vi "WPI_Power Get 3Volt Rail Voltage and Current.vi"(11 "error in":errorcluster) -> (6 "3.3 volt rail voltage (V)":dbl, 8 "3.3 volt rail current (A)":dbl, 15 "error out":errorcluster)   [LabVIEW 2017]
doc: "Returns the voltage and current of the 3.3 volt user rail on the roboRIO in the robot program. On the roboRIO the 3.3 volt rail is connected to:\npin V of DIO channels (internal jumper set to 3.3V)\npin 3.3V of SPI\npin 3.3V of I2C\npin 33 of MXP"
uses:
  <vilib>/Utility/error.llb/Error Cluster From Error Code.vi
  <vilib>/rvi/errors/niLvFpgaAdjustHostInterfaceError.vi
  <vilib>/rvi/interface/nirviReadWriteControl/nirviReadWriteControl.xnode
  <vilib>/Rock Robotics/SystemInterfaces/System/FPGA_SystemFRC FPGA Ref.ctl
  NiFpgaLv.dll
  <vilib>/rvi/interface/Simulation/niFpgaSimulationCallBeginRW.vi
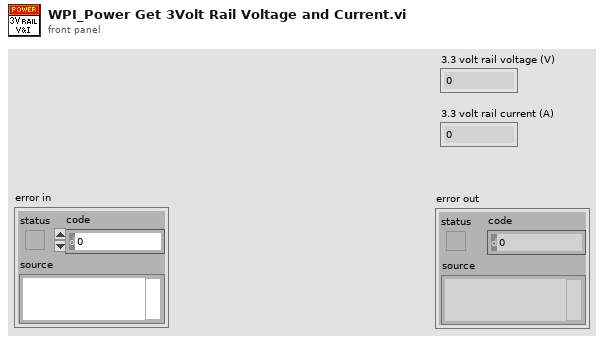
[diagram p1: front panel]
types:
  T1 = typedef "FPGA_SystemFRC FPGA Ref.ctl" = refnum<k20>
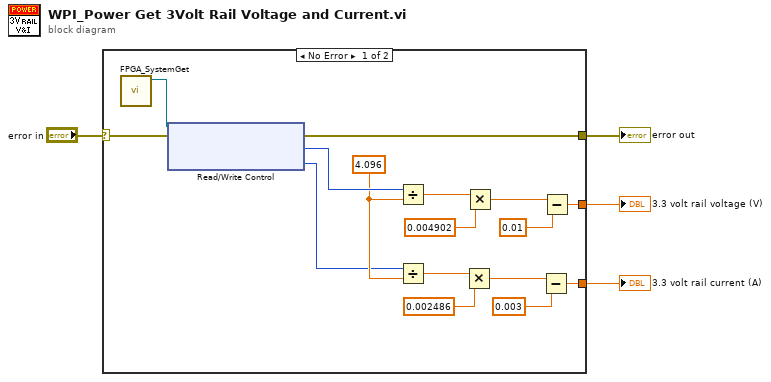
[diagram p0: block diagram]
diagram:
  n1 = case shown="No Error" "error in" {
    selector: "error in" -> [w6 w21]
    tunnel: [w5 w21] -> w3
    tunnel: [w17 _] -> w2
    tunnel: [w13 _] -> w1
    frame No Error {
      w10 = 4.096 ("battery voltage out")
      n2 = call <vilib>:"FPGA_SystemGet.vi"() -> ("FRC FPGA Ref"=w11:T1)  [unwired: 2 in, 9 out]
      n3 = xnode "Read/Write Control"("FPGA VI Reference In"=w11, "error in"=w6) -> ("error out"=w5:errorcluster, "Power.UserVoltage3V3"=w12:u16, "Power.UserCurrent3V3"=w9:u16)  [unwired: 1 out]
      n4 = Divide(x=w12, y=w10) -> (x/y=w7:dbl)
      n5 = Divide(x=w9, y=w10) -> (x/y=w8:dbl)
      n6 = Multiply(x=w8, y=0.002486 ("battery voltage out")) -> (x*y=w15:dbl)
      n7 = Multiply(x=w7, y=0.004902 ("battery voltage out")) -> (x*y=w19:dbl)
      n8 = Subtract(x=w15, y=0.003 ("battery voltage out")) -> (x-y=w13:dbl)
      n9 = Subtract(x=w19, y=0.01 ("battery voltage out")) -> (x-y=w17:dbl)
    }
    frame Error {
    }
  }
  "error out" <- w3
  "3.3 volt rail voltage (V)" <- w2
  "3.3 volt rail current (A)" <- w1
